vi "TDT-Run Circuit.vi"(11 "error in (no error)":errorcluster) -> (15 "error out":errorcluster)   [LabVIEW 2020]
uses:
  TDT-Globals.vi
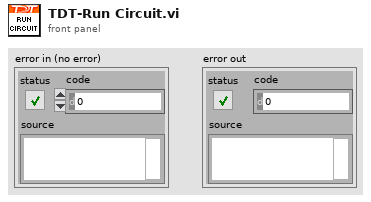
[diagram p1: front panel]
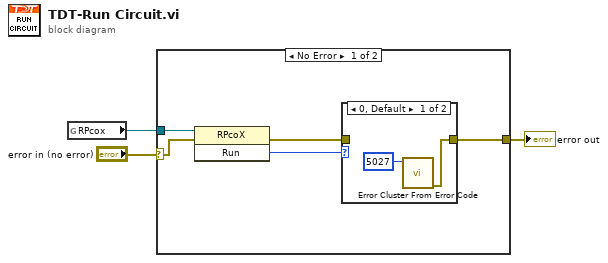
[diagram p0: block diagram]
diagram:
  n1 = global read "TDT-Globals.vi" "RPcox"() -> (w3:refnum<k7>)
  n2 = case shown="No Error" "error in (no error)" {
    selector: "error in (no error)" -> [w7 w12]
    tunnel: w3 -> [w8 _]
    tunnel: [w5 w12] -> w1
    frame No Error {
      n3 = invoke class="RPcoX" method="Run"(reference=w8, error in=w7) -> (error out=w4:errorcluster, "Run"=w6:i32)  [unwired: 1 in, 1 out]
      n4 = case shown="0, Default" w6 {
        tunnel: w4 -> [_ w11]
        tunnel: [w9 w11] -> w5
        frame 0, Default {
          n5 = call <vilib>:"Error Cluster From Error Code.vi"("error code (0)"=5027) -> ("error out"=w9:errorcluster)  [unwired: 8 in]
        }
        frame 1 {
        }
      }
    }
    frame Error {
    }
  }
  "error out" <- w1
